vi "Sub VI tutorial.vi"(11 "Temp F":dbl) -> (3 "Temp C":dbl)   [LabVIEW 2018]
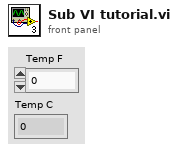
[diagram p1: front panel]
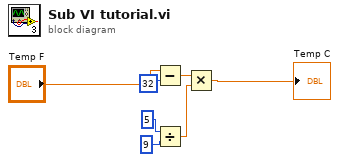
[diagram p0: block diagram]
diagram:
  n1 = Subtract(x="Temp F", y=32) -> (x-y=w4:dbl)
  n2 = Divide(x=5, y=9) -> (x/y=w3:dbl)
  n3 = Multiply(x=w4, y=w3) -> (x*y=→"Temp C":dbl)
